vi "Send Configure Standard Waveform [STD].vi"(2 "waveform (Sine)":i32(ring)=1 items=["Sine"=1, "Square"=2, "Triangle"=3, "Ramp Up"=4, "Ramp Down"=5, "DC"=6], 4 "amplitude (1.00 V)":dbl[unit]=1.0 format="%.3f", 5 "channel name (\"CHANNEL1\")":string="CHANNEL1", 6 "dc offset (0.00 V)":dbl[unit] format="%.3f", 7 "Message Priority (Normal)":T1=enum."Normal", 8 "error in (no error)":errorcluster, 9 "frequency (1000.0 Hz)":dbl[unit]=1000.0 format="%^.2e", 10 "start phase (0.00 Degrees)":dbl[unit] format="%.3f", 11 "Message Enqueuer":refnum<class "Message Enqueuer.lvclass">) -> (0 "error out":errorcluster, 3 "Message Enqueuer out":refnum<class "Message Enqueuer.lvclass">)   [LabVIEW 2013, in "CS++Fgen.lvlib" / "Configure Standard Waveform [STD] Msg.lvclass"]
doc: "This VI sends the message to an actor."
uses:
  Configure Standard Waveform [STD] Msg.lvclass
  <vilib>/ActorFramework/Message Enqueuer/Message Enqueuer.lvclass
  <vilib>/ActorFramework/Message Enqueuer/Message Priority.ctl
  Configure Standard Waveform [STD] Msg.lvclass/Configure Standard Waveform [STD] Msg.ctl
  <vilib>/ActorFramework/Message Enqueuer/Message Enqueuer.lvclass/Message Enqueuer.ctl
  <vilib>/ActorFramework/Message Priority Queue/Priority Enqueue.vi
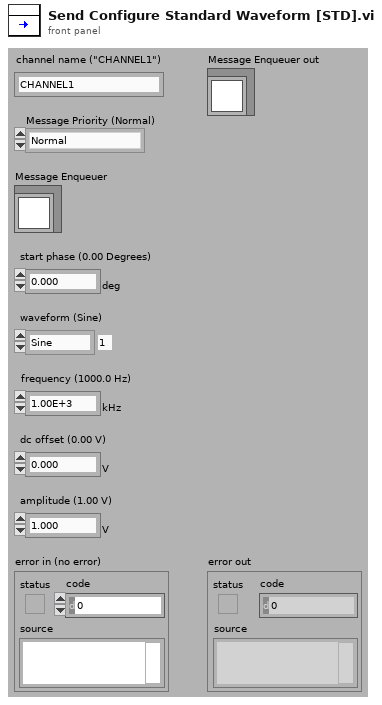
[diagram p1: front panel]
types:
  T1 = typedef "Actor Framework.lvlib/Message Enqueuer.lvclass/Message Priority.ctl" = enum16{"Low", "Normal", "High"}
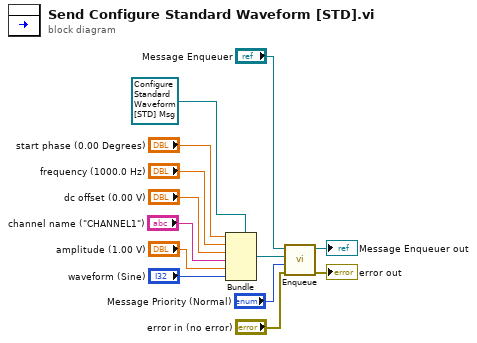
[diagram p0: block diagram]
diagram:
  n1 = Bundle(cluster=refnum<class "Configure Standard Waveform [STD] Msg.lvclass"> refnum ("Object"), "start phase (0.00 Degrees)", "frequency (1000.0 Hz)", "dc offset (0.00 V)", "channel name (\"CHANNEL1\")", "amplitude (1.00 V)", "waveform (Sine)") -> (w9:refnum<class "Configure Standard Waveform [STD] Msg.lvclass">)
  n2 = call <vilib>:"Enqueue.vi"("error in (no error)"="error in (no error)", "Message Priority (Normal)"="Message Priority (Normal)", "Message"=w9, "Message Enqueuer in"="Message Enqueuer") -> ("error out"=→"error out":errorcluster, "Message Enqueuer out"=→"Message Enqueuer out":refnum<class "Message Enqueuer.lvclass">)  [unwired: 6 in]
